vi "Format for dependency table.vi"(5 "# of Parent paths to remove in Path column":i32, 6 "Dependencies":T1[](array[typedef])) -> (2 "ItemNames":string[][](array[string]))   [LabVIEW 2013]
uses:
  Dependency cluster.ctl
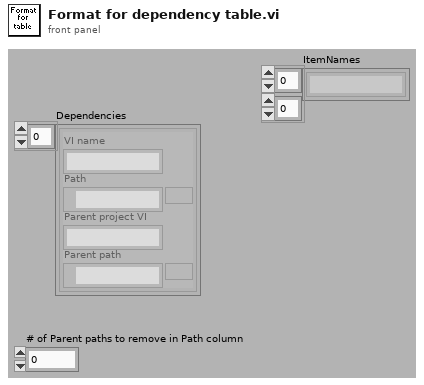
[diagram p1: front panel]
types:
  T1 = typedef "Dependency cluster.ctl" = cluster{"VI name":string, "Path":path, "Parent project VI":string, "Parent path":path}
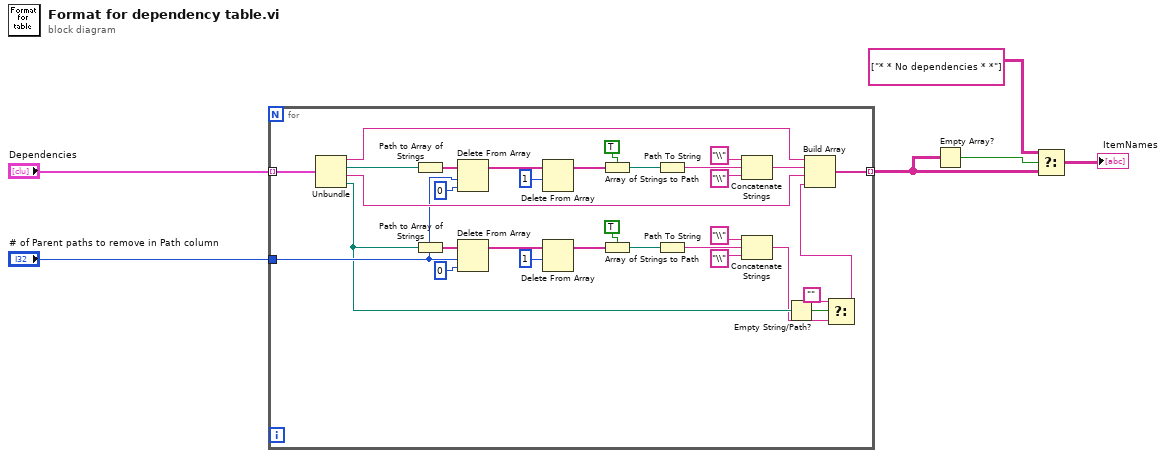
[diagram p0: block diagram]
diagram:
  n1 = for {
    tunnel: "Dependencies" -> [w38] mode=indexing
    tunnel: [w36] -> w6 mode=indexing
    tunnel: "# of Parent paths to remove in Path column" -> [w12]
    n2 = Unbundle(w38) -> ("VI name"=w37:string, "Path"=w33:path, "Parent project VI"=w30:string, "Parent path"=w11:path)
    n3 = Path to Array of Strings(0:w33) -> (2:w35:string[])  [unwired: 1 out]
    n4 = Path to Array of Strings(0:w11) -> (2:w13:string[])  [unwired: 1 out]
    n5 = Delete From Array(array=w35, length=w12, index=0) -> (array with subset deleted=w29:string[])  [unwired: 1 out]
    n6 = Delete From Array(array=w13, length=w12, index=0) -> (array with subset deleted=w17:string[])  [unwired: 1 out]
    n7 = Delete From Array(array=w29, length=1) -> (array with subset deleted=w27:string[])  [unwired: 1 in, 1 out]
    n8 = Delete From Array(array=w17, length=1) -> (array with subset deleted=w19:string[])  [unwired: 1 in, 1 out]
    n9 = Array of Strings to Path(0:w27, 1:TRUE ("relative")) -> (2:w32:path)
    n10 = Array of Strings to Path(0:w19, 1:TRUE ("relative")) -> (2:w15:path)
    n11 = Path To String(path=w32) -> (string=w26:string)
    n12 = Path To String(path=w15) -> (string=w20:string)
    n13 = Concatenate Strings("\\" ("string"), w26, "\\" ("string")) -> (w25:string)
    n14 = Concatenate Strings("\\" ("string"), w20, "\\" ("string")) -> (w8:string)
    n15 = Empty String/Path?(string/path=w11) -> (empty?=w10:bool)
    n16 = Select(t="", s=w10, f=w8) -> (s? t:f=w7:string)
    n17 = Build Array(w37, w25, w30, w7) -> (w36:string[])
  }
  n18 = Empty Array?(array=w6) -> (empty?=w2:bool)
  n19 = Select(t=string[][] [["* * No dependencies * *"]], s=w2, f=w6) -> (s? t:f=→"ItemNames":string[][])
